vi "Set Inheritances.vi"(10 "Class Info":T1[](array[typedef]), 11 "Module Class Ref Map":variant) -> (3 "Module Class Ref Map Dup":variant)   [LabVIEW 2013]
uses:
  Data Structures/JSON/Class.ctl
  Data Structures/JSON/Enum.ctl
  Data Structures/JSON/Enum Value.ctl
  Data Structures/JSON/Method.ctl
  Data Structures/JSON/Param.ctl
  Data Structures/JSON/Property.ctl
  Param Writers/TypeConv/Action.ctl
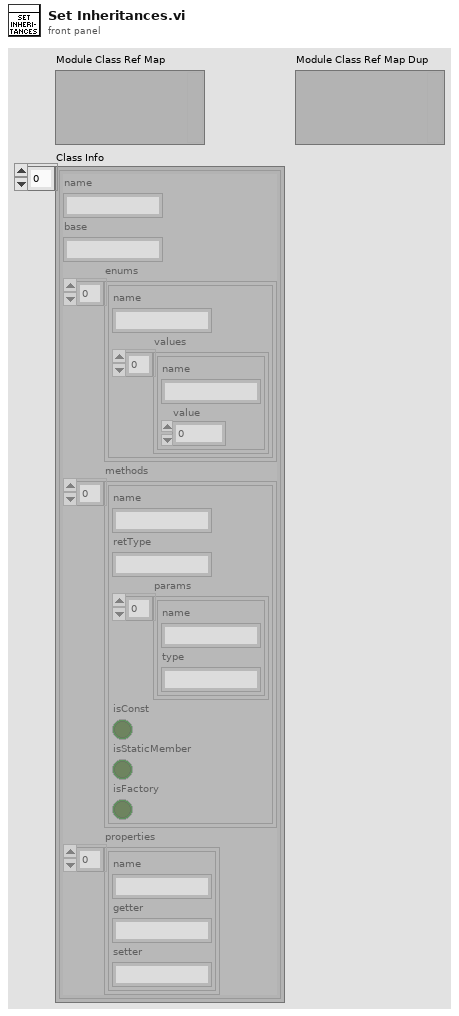
[diagram p1: front panel]
types:
  T1 = typedef "Class.ctl" = cluster{"name":string, "base":string, "enums":T2[], "methods":T4[], "properties":T6[]}
  T2 = typedef "Enum.ctl" = cluster{"name":string, "values":T3[]}
  T3 = typedef "Enum Value.ctl" = cluster{"name":string, "value":i32}
  T4 = typedef "Method.ctl" = cluster{"name":string, "retType":string, "params":T5[], "isConst":bool, "isStaticMember":bool, "isFactory":bool}
  T5 = typedef "Param.ctl" = cluster{"name":string, "type":string}
  T6 = typedef "Property.ctl" = cluster{"name":string, "getter":string, "setter":string}
  T7 = typedef "Action.ctl" = enum16{"Register Type", "Register Projection", "Obtain Writer", "Get Projection", "Get Type Path"}
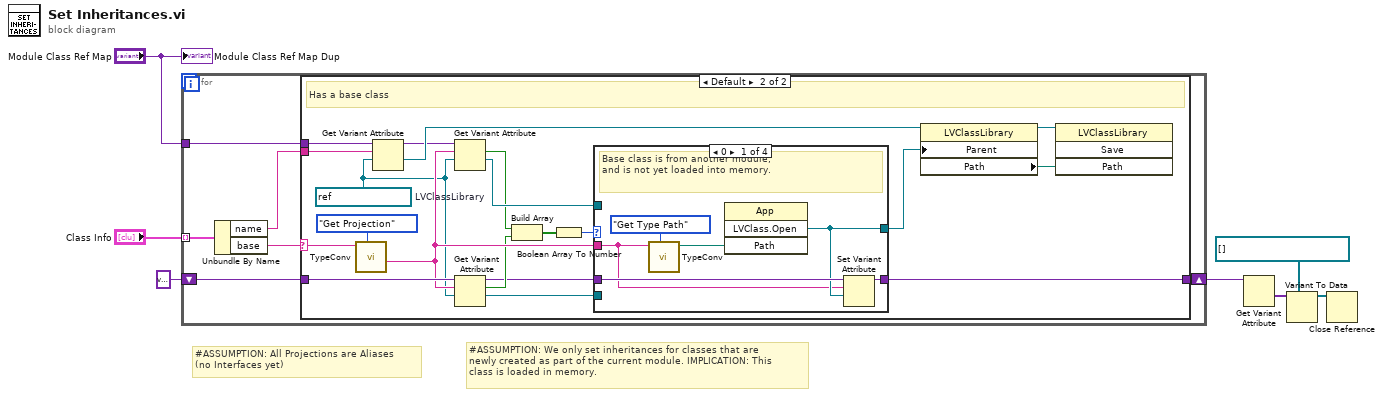
[diagram p0: block diagram]
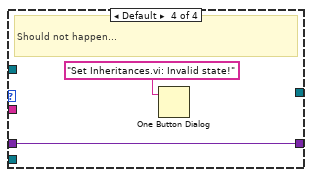
[diagram p5: hidden frame]
diagram:
  # "#ASSUMPTION: We only set inheritances for classes that are\nnewly created as part of the current module. IMPLICATION: This\nclass is loaded in memory."
  # "#ASSUMPTION: All Projections are Aliases\n(no Interfaces yet)"
  n1 = for {
    tunnel: "Class Info" -> [w13] mode=indexing
    tunnel: "Module Class Ref Map" -> [w12]
    shift-right: [w8] -> w4
    shift-left: variant ("Variant") -> [w9]
    n2 = Unbundle By Name(w13) -> ("name"=w10:string, "base"=w11:string)
    n3 = case shown="Default" w11 {
      selector: w11 -> [_ w27]
      tunnel: w12 -> [_ w31]
      tunnel: w10 -> [_ w30]
      tunnel: w9 -> [w14 w24]
      tunnel: [w14 w19] -> w8
      frame "" {
        # "Has no base class. No-op."
      }
      frame Default {
        w15 = refnum<vi> refnum  # LVClassLibrary
        # "Has a base class"
        n4 = call "TypeConv.vi"("Action"=Action."Get Projection", "Type Name"=w27) -> ("Projection Out"=w23:string)  [unwired: 6 in, 3 out]
        n5 = Get Variant Attribute(Variant=w31, name=w30, default value (empty Variant)=w15) -> (duplicate Variant=w26:variant, value=w29:refnum<vi>)  [unwired: 1 in, 2 out]
        n6 = Get Variant Attribute(Variant=w26, name=w23, default value (empty Variant)=w15) -> (found=w18:bool, value=w25:refnum<vi>)  [unwired: 1 in, 2 out]
        n7 = Get Variant Attribute(Variant=w24, name=w23, default value (empty Variant)=w15) -> (duplicate Variant=w20:variant, found=w22:bool, value=w16:refnum<vi>)  [unwired: 1 in, 1 out]
        n8 = Build Array(w18, w22) -> (w21:bool[])
        n9 = Boolean Array To Number(Boolean array=w21) -> (number=w17:u32)
        n10 = case shown="0" w17 {
          tunnel: w20 -> [w38 w42 w44 w45]
          tunnel: [w37 w41 w43 _] -> w28
          tunnel: [w36 w42 w44 w45] -> w19
          tunnel: w23 -> [w35 _ _ _]
          tunnel: w25 -> [_ w41 _ _]
          tunnel: w16 -> [_ _ w43 _]
          frame 0 {
            # "Base class is from another module,\nand is not yet loaded into memory."
            n11 = call "TypeConv.vi"("Action"=Action."Get Type Path", "Type Name"=w35) -> ("Type Path"=w39:path)  [unwired: 6 in, 3 out]
            n12 = invoke class="App" method="LVClass.Open"("Path"=w39) -> ("LVClass.Open"=w37:refnum<vi>)  [unwired: 3 in, 3 out]
            n13 = Set Variant Attribute(Variant=w38, name=w35, value=w37) -> (Variant out=w36:variant)  [unwired: 1 in, 2 out]
          }
          frame 1 {
            # "Base class is in the current module,\nand is therefore already in memory."
          }
          frame 2 {
            # "Base class is from another module,\nand is already in memory."
          }
          frame Default {
            # "Should not happen..."
            n14 = One Button Dialog(message="Set Inheritances.vi: Invalid state!") -> ()  [unwired: 1 in, 1 out]
          }
        }
        n15 = property class="LVClassLibrary"(reference=w29, "Parent"=w28) -> (reference out=w34:refnum<vi>, "Path"=w33:path)  [unwired: 1 in, 1 out]
        n16 = invoke class="LVClassLibrary" method="Save"(reference=w34, "Path"=w33) -> ()  [unwired: 2 in, 4 out]
      }
    }
  }
  n17 = Get Variant Attribute(Variant=w4) -> (values=w3:variant[])  [unwired: 3 in, 3 out]
  n18 = Variant To Data(type=refnum<vi>[] [], Variant=w3) -> (data=w1:refnum<vi>[])  [unwired: 1 in, 1 out]
  n19 = Close Reference(reference=w1) -> ()  [unwired: 1 in, 1 out]
  "Module Class Ref Map Dup" <- "Module Class Ref Map"
